vi "Interface Unit_Counter.vi"(3 "CI.CountEdges.Term":tag="/PXI-6624/PFI34", 5 "Counter Physical Channel":tag="PXI-6624/ctr1") -> (0 "error out":errorcluster, 1 "CI.CountEdges.Dir":i32(ring)=10128 items=["Count Up"=10128, "Count Down"=10124, "Externally Controlled"=10326], 2 "data":dbl[](array[numeric]) format="%0.2f")   [LabVIEW 2019, in "SubVIs.lvlib" / "Tachometer VI.lvlib"]
uses:
  Tachometer VI.lvlib
  <vilib>/DAQmx/read.llb/DAQmx Read (Counter 1D DBL 1Chan NSamp).vi
  <vilib>/DAQmx/create/channels.llb/DAQmx Create Channel (CI-Count Edges).vi
  <vilib>/DAQmx/miscellaneous.llb/DAQmx Fill In Error Info.vi
  <resource>/objmgr/daqmx.rc
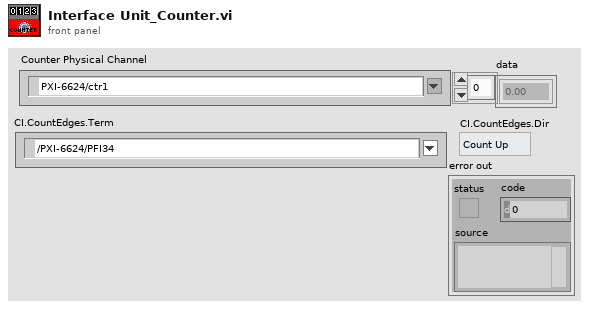
[diagram p1: front panel]
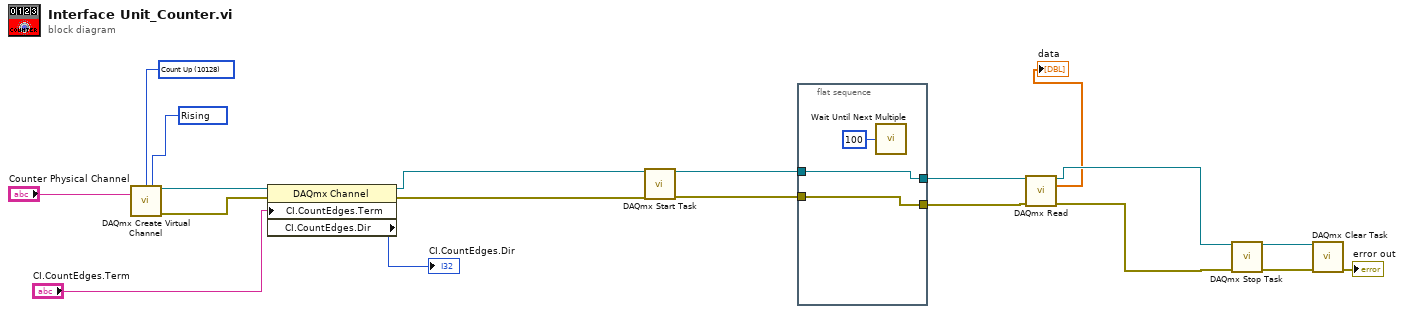
[diagram p0: block diagram]
diagram:
  w17 = 10280 items=["Rising"=10280, "Falling"=10171] ("edge")
  w18 = 10128 items=["Count Up"=10128, "Count Down"=10124, "Externally Controlled"=10326] ("count direction")
  n1 = call-poly <vilib>:"DAQmx Create Virtual Channel.vi"("count direction"=w18, "edge"=w17, "counter"="Counter Physical Channel") -> ("task out"=w15:refnum<k21>, "error out"=w16:errorcluster)  [unwired: 11 in]
  n2 = property class="DAQmx Channel"(reference=w15, error in=w16, "CI.CountEdges.Term"="CI.CountEdges.Term") -> (reference out=w12:refnum<k21>, error out=w11:errorcluster, "CI.CountEdges.Dir"=→"CI.CountEdges.Dir":i32)
  n3 = call <vilib>:"DAQmx Start Task.vi"("task/channels in"=w12, "error in"=w11) -> ("task out"=w4:refnum<k21>, "error out"=w2:errorcluster)  [unwired: 12 in]
  n4 = flat-sequence {
    tunnel: [w22] -> w5
    tunnel: w4 -> [w22]
    tunnel: [w21] -> w3
    tunnel: w2 -> [w21]
    frame #0 {
      n5 = call "Wait Until Next Multiple"("Count(mSec)"=u32 100) -> ()  [unwired: 1 out]
    }
  }
  n6 = call-poly <vilib>:"DAQmx Read.vi"("task/channels in"=w5, "error in"=w3) -> ("task out"=w10:refnum<k21>, "data"=→"data":dbl[], "error out"=w9:errorcluster)  [unwired: 11 in]
  n7 = call <vilib>:"DAQmx Stop Task.vi"("task/channels in"=w10, "error in"=w9) -> ("task out"=w14:refnum<k21>, "error out"=w13:errorcluster)  [unwired: 12 in]
  n8 = call <vilib>:"DAQmx Clear Task.vi"("task in"=w14, "error in"=w13) -> ("error out"=→"error out":errorcluster)  [unwired: 13 in]
